vi "get Node Position in subBranch.vi"(8 "error in (no error)":errorcluster, 11 "xceDataNode in":refnum<class "xceDataNode.lvclass">) -> (0 "error out":errorcluster, 2 "Position":string, 3 "xceDataNode out":refnum<class "xceDataNode.lvclass">)   [LabVIEW 2013, in "xceDataNode.lvclass"]
uses:
  xceDataNode.lvclass
  xceNode/xceNode.lvclass
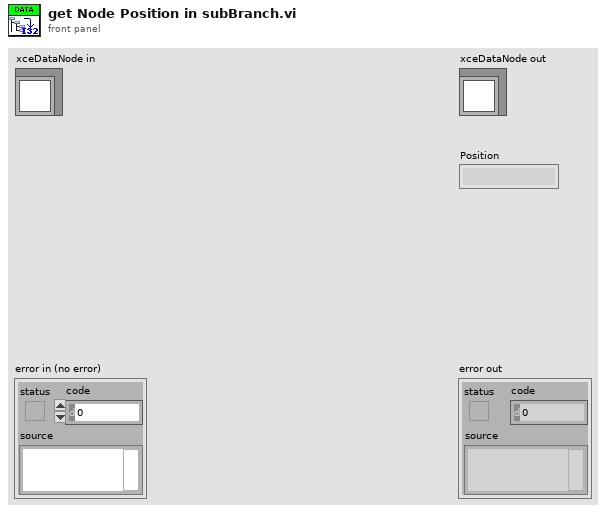
[diagram p1: front panel]
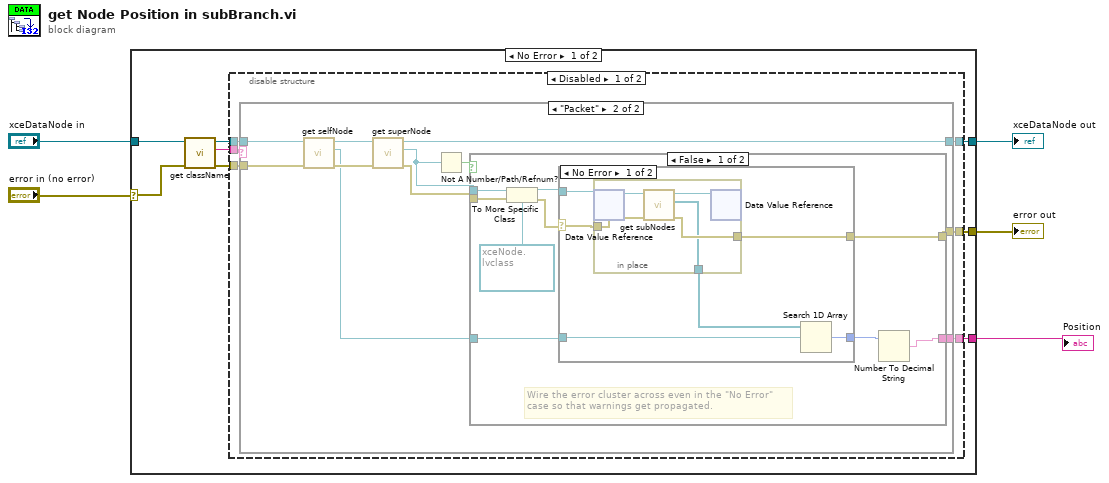
[diagram p0: block diagram]
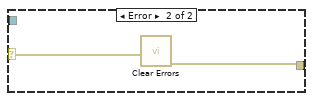
[diagram p3: hidden frame]
diagram:
  n1 = case shown="No Error" "error in (no error)" {
    selector: "error in (no error)" -> [w9 w59]
    tunnel: [w11 w59] -> w4
    tunnel: [w13 w58] -> w2
    tunnel: "xceDataNode in" -> [w10 w58]
    tunnel: [w12 _] -> w1
    frame No Error {
      n2 = call "get className.vi"("error in (no error)"=w9, "xceNode in"=w10) -> ("error out"=w6:errorcluster, "Class name"=w7:string, "xceNode out"=w8:refnum<class "xceDataNode.lvclass">)  [unwired: 7 in]
      n3 = disable-structure shown="Disabled" {
        disable-tunnel: [w19 w57] -> w13
        disable-tunnel: [w18 _] -> w12
        disable-tunnel: [w17 w56] -> w11
        disable-tunnel: w8 -> [w16 w57]
        disable-tunnel: w7 -> [w15 _]
        disable-tunnel: w6 -> [w14 w56]
        frame Disabled {
          n4 = case shown="\"Packet\"" w15 {
            tunnel: [w21 w29] -> w19
            tunnel: [_ w27] -> w18
            tunnel: [w20 w26] -> w17
            tunnel: w16 -> [w21 w23]
            tunnel: w14 -> [w20 w22]
            frame Default {
            }
            frame "Packet" {
              n5 = call "get selfNode.vi"("error in (no error)"=w22, "xceNode in"=w23) -> ("error out"=w32:errorcluster, "selfNode*"=w28:refnum<data-value>, "xceNode out"=w31:refnum<class "xceDataNode.lvclass">)  [unwired: 7 in]
              n6 = call "get superNode.vi"("error in (no error)"=w32, "xceNode in"=w31) -> ("error out"=w30:errorcluster, "superNode*"=w25:refnum<data-value>, "xceNode out"=w29:refnum<class "xceDataNode.lvclass">)  [unwired: 7 in]
              n7 = Not A Number/Path/Refnum?(number/path/refnum=w25) -> (NaN/Path/Refnum?=w24:bool)
              n8 = case shown="False" w24 {
                tunnel: w30 -> [w39 w55]
                tunnel: w28 -> [w38 _]
                tunnel: [w33 _] -> w27
                tunnel: [w36 w55] -> w26
                tunnel: w25 -> [w35 _]
                frame False {
                  # "Wire the error cluster across even in the \"No Error\"\ncase so that warnings get propagated."
                  n9 = To More Specific Class(target class=refnum<data-value> refnum ("data value reference"), reference=w35, error in=w39) -> (specific class reference=w41:refnum<data-value>, error out=w37:errorcluster)
                  n10 = case shown="No Error" w37 {
                    selector: w37 -> [w43 w54]
                    tunnel: w41 -> [w47 _]
                    tunnel: w38 -> [w45 _]
                    tunnel: [w44 _] -> w34
                    tunnel: [w42 w53] -> w36
                    frame No Error {
                      n11 = in-place {
                        in-place-border: w43 -> [w51]
                        in-place-border: [w49] -> w42
                        in-place-border: [w48] -> w46
                        n12 = in-place-dvr #1(w47) -> (w52:refnum<class "xceNode.lvclass">)  [unwired: 1 out]
                        n13 = call "get subNodes.vi"("error in (no error)"=w51, "xceNode in"=w52) -> ("error out"=w49:errorcluster, "subNodes[]*"=w48:refnum<data-value>[], "xceNode out"=w50:refnum<class "xceNode.lvclass">)  [unwired: 7 in]
                        n14 = in-place-dvr #1(w50) -> ()  [unwired: 2 out]
                      }
                      n15 = Search 1D Array(1D array=w46, element=w45) -> (index of element=w44:i32)  [unwired: 1 in]
                    }
                    frame Error {
                      n16 = call <vilib>:"Clear Errors.vi"("error in (no error)"=w54) -> ("error out"=w53:errorcluster)  [unwired: 6 in]
                    }
                  }
                  n17 = Number To Decimal String(number=w34) -> (decimal integer string=w33:string)  [unwired: 1 in]
                }
                frame True {
                }
              }
            }
          }
        }
        frame Enabled {
        }
      }
    }
    frame Error {
    }
  }
  "error out" <- w4
  "xceDataNode out" <- w2
  "Position" <- w1
